vi "Main.vi"(11 "Module Admin":refnum<class "Delacor_lib_QMH_Module Admin.lvclass">) -> ()   [LabVIEW 2019, in "UI.lvlib"]
doc: "This template is based off of the Queued Message Handler design pattern and the Queued Message Handler project template that ships with LabVIEW.\n\nThe main difference is that the queue is private to this module and communication between modules is performed via Broadcast and Request events.\n\nRequest events are wrapped in public API methods and are handled in the Event Handling Loop (EHL) of this VI. Any module can register for Broadcast events sent by this module. The EHL generates messages based on user interface actions.\n\nThe Message Handling Loop (MHL) processes messages generated by the EHL, or by other messages. The messages are string values, so new messages can be added easily to the Message Cases case structure in the MHL. Each message cluster can also provide an optional value for Message Data, which is a variant that can be converted to whatever message-specific data is required.\n_____\nBased on Delacor QMH Project Template 5.0.0.82."
uses:
  UI.lvlib
  <vilib>/Delacor/Delacor QMH/Libraries/Module Admin_class/Delacor_lib_QMH_Module Admin.lvclass
  Module Data--cluster.ctl
  Stop Argument--cluster.ctl
  <vilib>/Delacor/Delacor QMH/Libraries/Message Queue_class/Delacor_lib_QMH_Message Queue.lvclass/Delacor_lib_QMH_Message Queue.ctl
  <vilib>/Delacor/Delacor QMH/Libraries/Module Admin_class/Delacor_lib_QMH_Module Admin.lvclass/Delacor_lib_QMH_Module Admin.ctl
  <vilib>/Delacor/Delacor QMH/Libraries/Message Queue_class/Delacor_lib_QMH_Enqueue Message (Single).vi
  <vilib>/Delacor/Delacor QMH/Libraries/Module Admin_class/Delacor_lib_QMH_Get External Launch.vi
  <vilib>/Utility/error.llb/Error Cluster From Error Code.vi
  <vilib>/ErrorRing/Error Ring.xnode
  <vilib>/Delacor/Delacor QMH/Libraries/Message Queue_class/Delacor_lib_QMH_Message Queue.lvclass
  Mensajes/Messages.lvlib
  Monedas/Monedas.lvlib
  Products/Products.lvlib
  Configuration/Configuration.lvlib
panel:
  out "error out":errorcluster
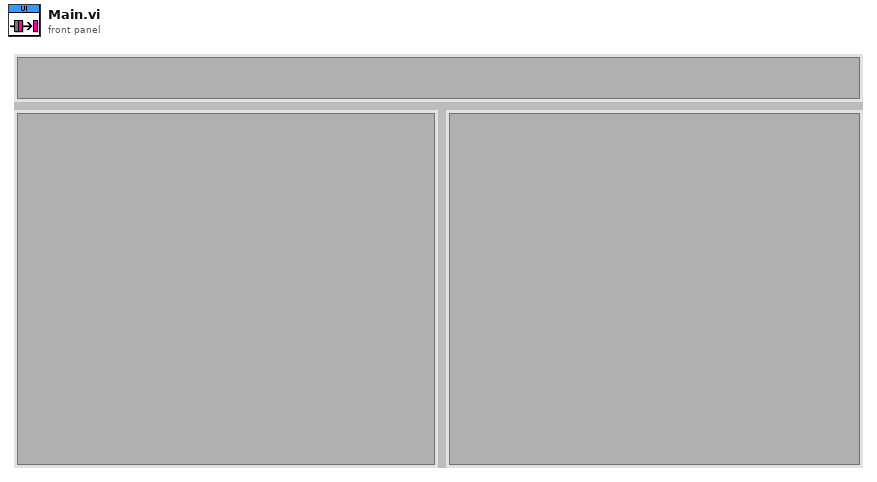
[diagram p1: front panel]
types:
  T1 = typedef "UI.lvlib/Request Events--cluster.ctl" = cluster{"Stop Module":refnum<user-event>, "Show Panel":refnum<user-event>, "Hide Panel":refnum<user-event>, "Get Module Execution Status":refnum<user-event>, "Show Diagram":refnum<user-event>}
  T2 = typedef "Messages.lvlib/Broadcast Events--cluster.ctl" = cluster{"Module Did Init":refnum<user-event>, "Status Updated":refnum<user-event>, "Error Reported":refnum<user-event>, "Module Did Stop":refnum<user-event>, "Update Module Execution Status":refnum<user-event>}
  T3 = typedef "Monedas.lvlib/Broadcast Events--cluster.ctl" = cluster{"Module Did Init":refnum<user-event>, "Status Updated":refnum<user-event>, "Error Reported":refnum<user-event>, "Module Did Stop":refnum<user-event>, "Update Module Execution Status":refnum<user-event>}
  T4 = typedef "Products.lvlib/Broadcast Events--cluster.ctl" = cluster{"Module Did Init":refnum<user-event>, "Status Updated":refnum<user-event>, "Error Reported":refnum<user-event>, "Module Did Stop":refnum<user-event>, "Update Module Execution Status":refnum<user-event>}
  T5 = typedef "Configuration.lvlib/Broadcast Events--cluster.ctl" = cluster{"Module Did Init":refnum<user-event>, "Status Updated":refnum<user-event>, "Error Reported":refnum<user-event>, "Module Did Stop":refnum<user-event>, "Update Module Execution Status":refnum<user-event>}
  T6 = typedef "UI.lvlib/Module Data--cluster.ctl" = cluster{"Status":string}
  T7 = enum32{"invalid lock state", "Not Locked", "Locked (No Password)", "Password-protected"}
  T8 = typedef "UI.lvlib/Stop Argument--cluster.ctl" = cluster{"Origin":string, "Exit via Stop Module Req?":bool, "Wait for Module to stop?":bool}
  T9 = enum32{"Invalid", "Standard", "Closed", "Hidden", "Minimized", "Maximized"}
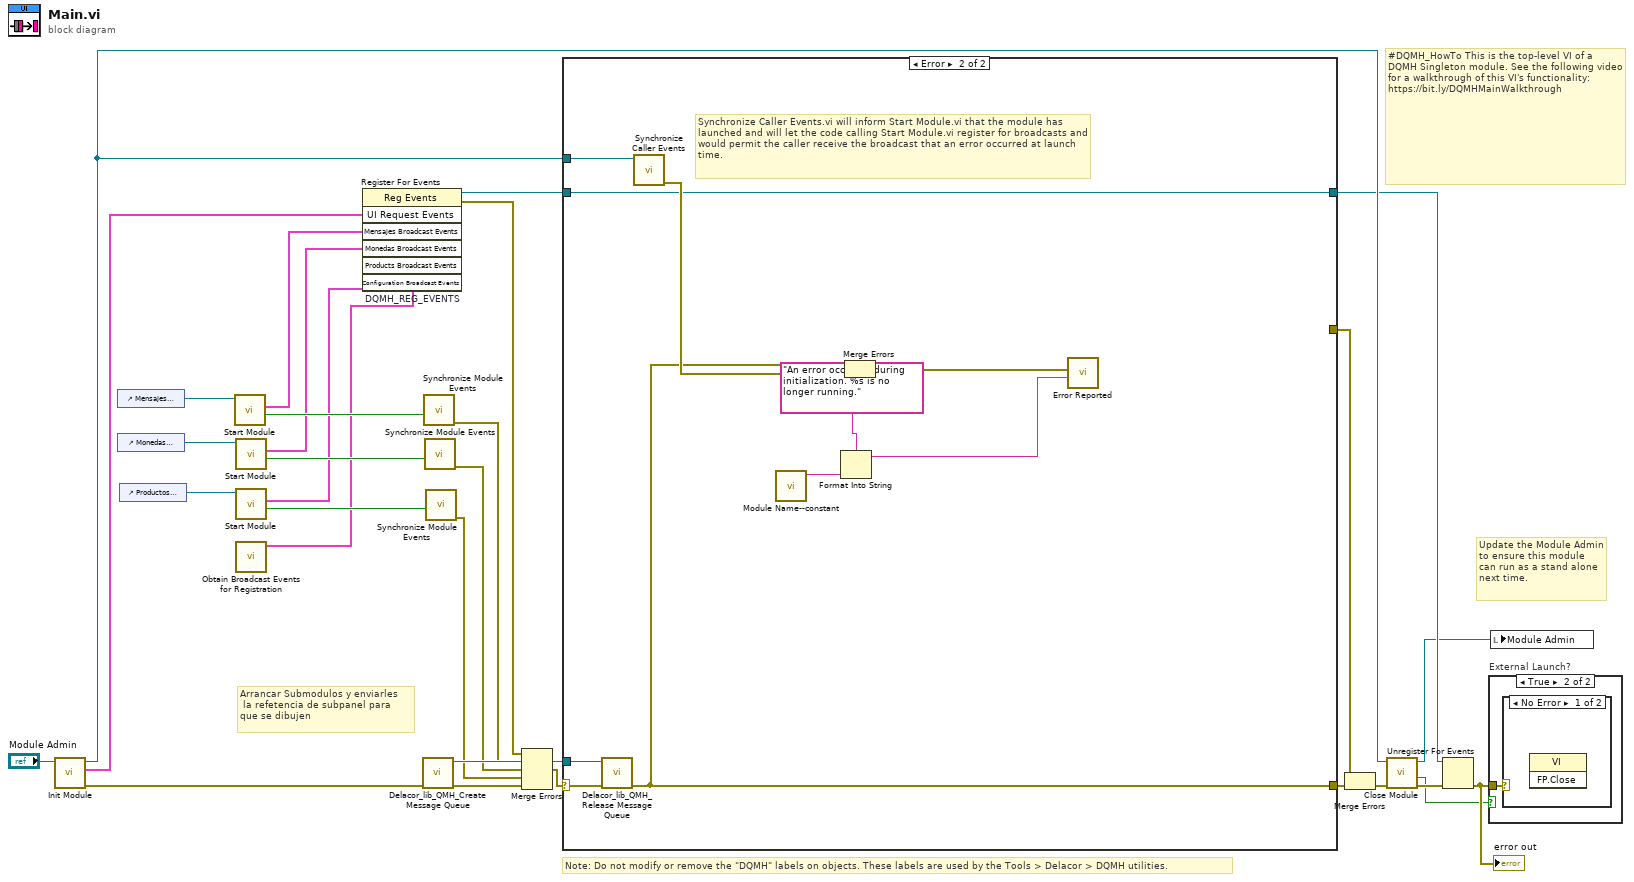
[diagram p0: block diagram]
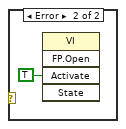
[diagram p3: hidden frame]
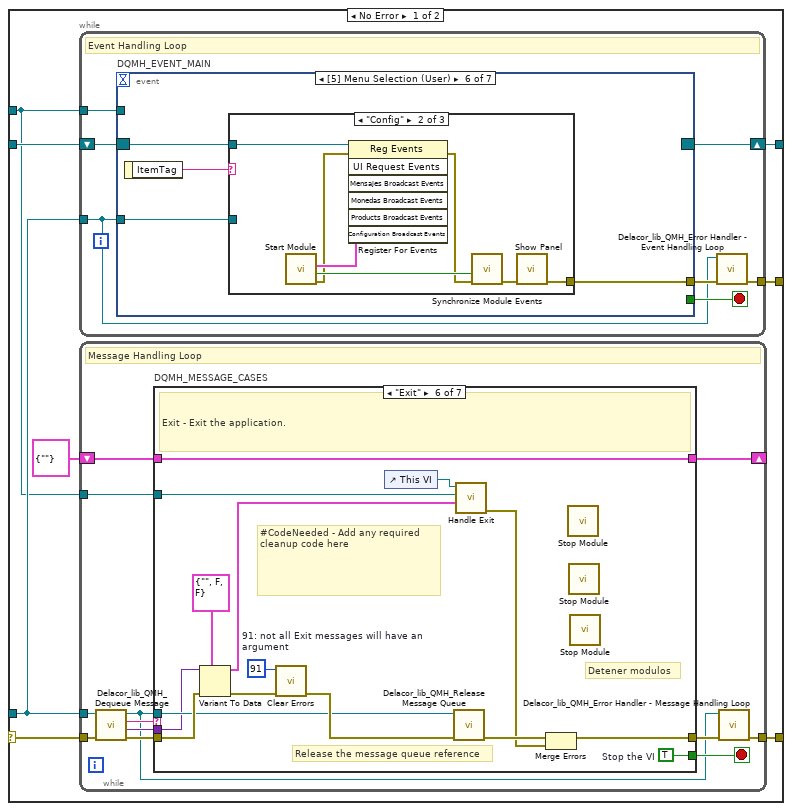
[diagram p4: hidden frame]
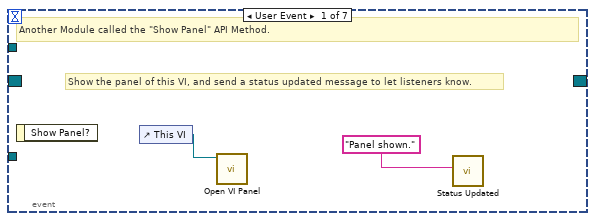
[diagram p5: hidden frame]
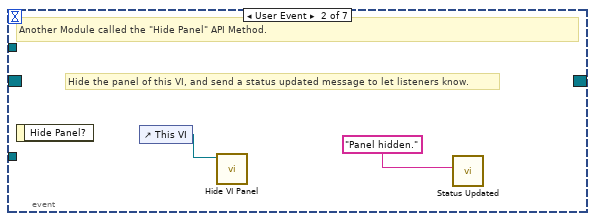
[diagram p6: hidden frame]
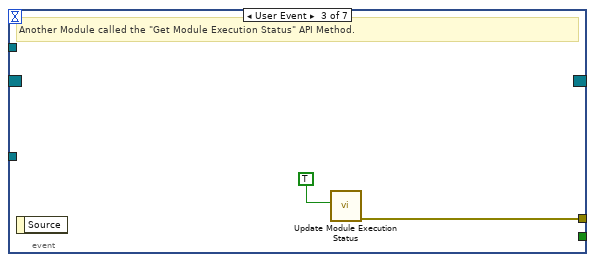
[diagram p7: hidden frame]
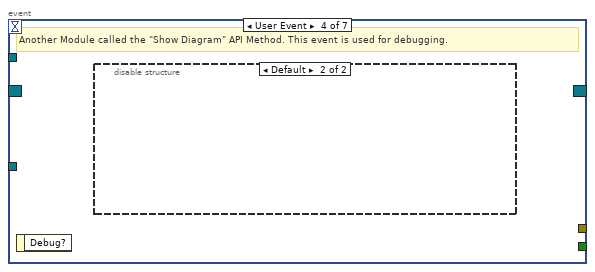
[diagram p8: hidden frame]
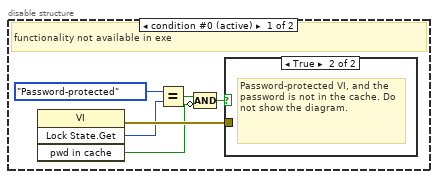
[diagram p9: hidden frame]
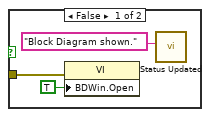
[diagram p10: hidden frame]
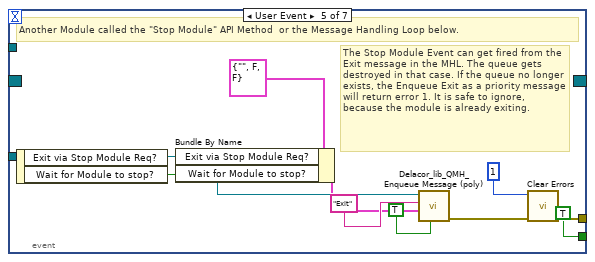
[diagram p11: hidden frame]
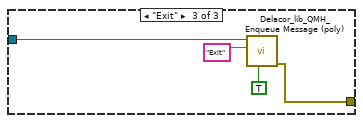
[diagram p13: hidden frame]
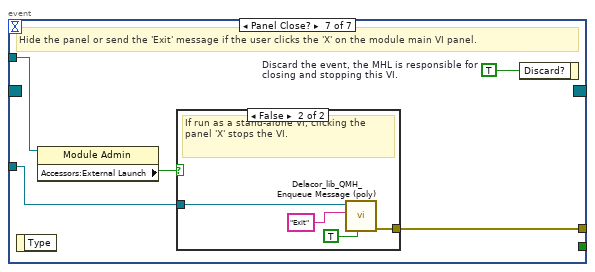
[diagram p14: hidden frame]
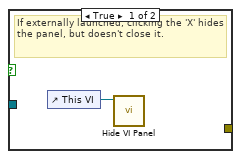
[diagram p15: hidden frame]
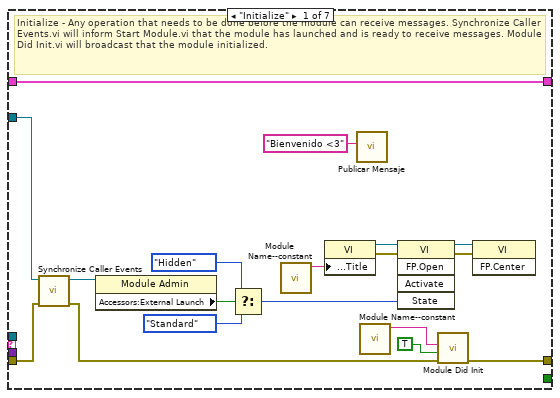
[diagram p16: hidden frame]
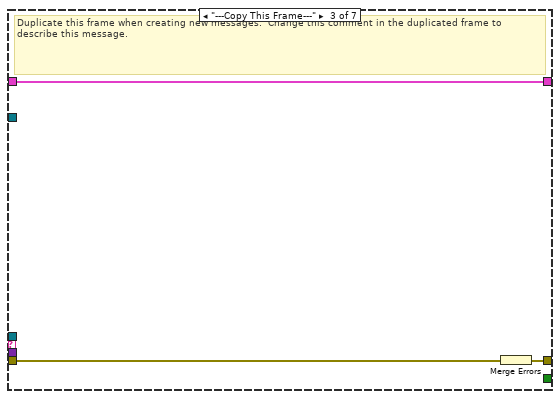
[diagram p18: hidden frame]
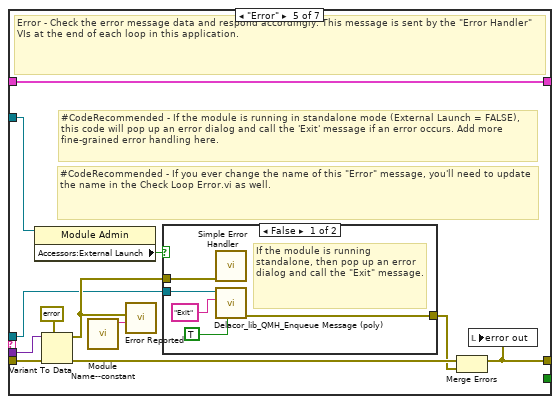
[diagram p20: hidden frame]
diagram:
  # "Arrancar Submodulos y enviarles\n la refetencia de subpanel para \nque se dibujen"
  # "#DQMH_HowTo This is the top-level VI of a DQMH Singleton module. See the following video for a walkthrough of this VI's functionality: https://bit.ly/DQMHMainWalkthrough"
  # "Note: Do not modify or remove the \"DQMH\" labels on objects. These labels are used by the Tools > Delacor > DQMH utilities."
  # "Update the Module Admin to ensure this module can run as a stand alone next time."
  n1 = call "Init Module.vi"("Singleton Module Admin in"="Module Admin") -> ("error out"=w29:errorcluster, "UI Request Events"=w19:T1, "Singleton Module Admin out"=w22:refnum<class "Delacor_lib_QMH_Module Admin.lvclass">)  [unwired: 8 in]
  n2 = control-ref of="Mensajes Subpanel"() -> (w11:refnum<vi>)
  n3 = control-ref of="Monedas Subpanel"() -> (w3:refnum<vi>)
  n4 = control-ref of="Productos Subpanel"() -> (w2:refnum<vi>)
  n5 = call "Start Module.vi"("Mensajes Subpanel"=w11) -> ("Wait for Event Sync?"=w14:bool, "Mensajes Broadcast Events"=w10:T2)  [unwired: 7 in, 2 out]
  n6 = call "Start Module.vi"("Monedas Subpanel"=w3) -> ("Wait for Event Sync?"=w13:bool, "Monedas Broadcast Events"=w9:T3)  [unwired: 7 in, 2 out]
  n7 = call "Start Module.vi"("Productos Subpanel"=w2) -> ("Wait for Event Sync?"=w12:bool, "Products Broadcast Events"=w8:T4)  [unwired: 7 in, 2 out]
  n8 = call "Obtain Broadcast Events for Registration.vi"() -> ("Configuration Broadcast Events"=w1:T5)  [unwired: 9 in, 2 out]
  n9 = register-events "DQMH_REG_EVENTS"(w19, w10, w9, w8, w1) -> (reference out=w20:refnum<event-registration>, error out=w4:errorcluster)  [unwired: 2 in]
  n10 = call <vilib>:"Delacor_lib_QMH_Create Message Queue.vi"("error in (no error)"=w29) -> ("error out"=w24:errorcluster, "Message Queue"=w18:refnum<class "Delacor_lib_QMH_Message Queue.lvclass">)  [unwired: 9 in]
  n11 = call "Synchronize Module Events.vi"("Wait for Event Sync?"=w14) -> ("error out"=w5:errorcluster)  [unwired: 10 in]
  n12 = call "Synchronize Module Events.vi"("Wait for Event Sync?"=w13) -> ("error out"=w6:errorcluster)  [unwired: 10 in]
  n13 = call "Synchronize Module Events.vi"("Wait for Event Sync?"=w12) -> ("error out"=w7:errorcluster)  [unwired: 10 in]
  n14 = Merge Errors(w4, w5, w6, w7, w24) -> (w23:errorcluster)
  n15 = case shown="Error" w23 {
    selector: w23 -> [w36 w182]
    tunnel: [w38 w181] -> w30
    tunnel: [w35 w187] -> w21
    tunnel: w20 -> [w33 w187]
    tunnel: w18 -> [w32 w180]
    tunnel: [w37 _] -> w27
    tunnel: w22 -> [w31 w183]
    frame No Error {
      n16 = while {
        tunnel: w32 -> [w39]
        shift-right: [w42] -> w35
        shift-left: w33 -> [w43]
        tunnel: [w44] -> w37
        tunnel: w31 -> [w40]
        stop <- w41 stop-if-true
        # "Event Handling Loop"
        n17 = event "DQMH_EVENT_MAIN" shown="[5] Menu Selection (User)" {
          selector: w43 -> [_ _ _ _ _ w73 _]
          dyn-events: [_ _ _ _ _ _ _] -> w42
          timeout: _ -> [_ _ _ _ _ _ _]
          tunnel: [_ _ _ _ TRUE ("Discard?") _ _] -> w41
          tunnel: w39 -> [_ _ _ _ w67 w74 w89]
          tunnel: [_ _ w51 _ w70 w72 w91] -> w45
          tunnel: w40 -> [_ _ _ _ _ _ w88]
          event User Event {
            # "Show the panel of this VI, and send a status updated message to let listeners know."
            # "Another Module called the \"Show Panel\" API Method."
            n18 = event-data() -> ()  [unwired: 1 in, 1 out]
            n19 = control-ref of="This VI"() -> (w47:refnum<vi>)
            n20 = call "Open VI Panel.vi"("VI"=w47) -> ()  [unwired: 10 in, 1 out]
            n21 = call "Status Updated.vi"("Status"="Panel shown." ("format string")) -> ()  [unwired: 10 in, 1 out]
          }
          event User Event {
            # "Hide the panel of this VI, and send a status updated message to let listeners know."
            # "Another Module called the \"Hide Panel\" API Method."
            n22 = event-data() -> ()  [unwired: 1 in, 1 out]
            n23 = control-ref of="This VI"() -> (w49:refnum<vi>)
            n24 = call "Hide VI Panel.vi"("VI"=w49) -> ()  [unwired: 10 in, 1 out]
            n25 = call "Status Updated.vi"("Status"="Panel hidden." ("format string")) -> ()  [unwired: 10 in, 1 out]
          }
          event User Event {
            # "Another Module called the \"Get Module Execution Status\" API Method."
            n26 = event-data() -> ()  [unwired: 1 in, 1 out]
            n27 = call "Update Module Execution Status.vi"("Running?"=TRUE) -> ("error out"=w51:errorcluster)  [unwired: 10 in]
          }
          event User Event {
            # "Another Module called the \"Show Diagram\" API Method. This event is used for debugging."
            n28 = event-data() -> ()  [unwired: 1 in, 1 out]
            n29 = disable-structure shown="Default" {
              frame condition #0 (active) {
                # "functionality not available in exe"
                n30 = invoke class="VI" method="Lock State.Get"() -> (error out=w57:errorcluster, "Get Lock State"=w56:T7, "pwd in cache"=w53:bool)  [unwired: 4 in, 1 out]
                n31 = Equal?(x=T7."Password-protected", y=w56) -> (x = y?=w54:bool)
                n32 = Compound Arithmetic op=AND(w54, invert w53) -> (w52:bool)
                n33 = case shown="True" w52 {
                  tunnel: w57 -> [w60 _]
                  frame False {
                    n34 = property class="VI"(error in=w60, "BDWin.Open"=TRUE ("Block Diagram Window:Open")) -> ()  [unwired: 1 in, 2 out]
                    n35 = call "Status Updated.vi"("Status"="Block Diagram shown." ("format string")) -> ()  [unwired: 10 in, 1 out]
                  }
                  frame True {
                    # "Password-protected VI, and the password is not in the cache. Do not show the diagram."
                  }
                }
              }
              frame condition #1 {
              }
            }
          }
          event User Event {
            # "The Stop Module Event can get fired from the Exit message in the MHL. The queue gets destroyed in that case. If the queue no longer exists, the Enqueue Exit as a priority message will return error 1. It is safe to ignore, because the module is already exiting."
            # "Another Module called the \"Stop Module\" API Method  or the Message Handling Loop below."
            n36 = event-data() -> ("Exit via Stop Module Req?"=w63:bool, "Wait for Module to stop?"=w62:bool)  [unwired: 1 in]
            n37 = Bundle By Name(cluster=T8 {"Origin"="", "Exit via Stop Module Req?"=FALSE, "Wait for Module to stop?"=FALSE} ("Stop Argument"), "Exit via Stop Module Req?"=w63, "Wait for Module to stop?"=w62) -> (w61:T8)
            n38 = call-poly <vilib>:"Delacor_lib_QMH_Enqueue Message (poly).vi"("Priority Message? (F)"=TRUE, "Message Data"=w61, "Message"="Exit", "Message Queue in"=w67) -> ("error out"=w71:errorcluster)  [unwired: 6 in, 1 out]
            n39 = call <vilib>:"Clear Errors.vi"("error in (no error)"=w71, "specific error code to clear (0: all)"=1) -> ("error out"=w70:errorcluster)  [unwired: 4 in, 1 out]
          }
          event Menu Selection (User) {
            n40 = event-data() -> ("ItemTag"=w75:string)  [unwired: 1 in]
            n41 = case shown="\"Config\"" w75 {
              tunnel: w74 -> [_ _ w84]
              tunnel: w73 -> [_ w82 _]
              tunnel: [_ w76 w83] -> w72
              frame "False", Default {
              }
              frame "Config" {
                n42 = call "Start Module.vi"() -> ("error out"=w79:errorcluster, "Wait for Event Sync?"=w80:bool, "Configuration Broadcast Events"=w81:T5)  [unwired: 8 in, 1 out]
                n43 = register-events(reference=w82, error in=w79, w81) -> (error out=w78:errorcluster)  [unwired: 4 in, 1 out]
                n44 = call "Synchronize Module Events.vi"("error in (no error)"=w78, "Wait for Event Sync?"=w80) -> ("error out"=w77:errorcluster)  [unwired: 9 in]
                n45 = call "Show Panel.vi"("error in (no error)"=w77) -> ("error out"=w76:errorcluster)  [unwired: 10 in]
              }
              frame "Exit" {
                n46 = call-poly <vilib>:"Delacor_lib_QMH_Enqueue Message (poly).vi"("Priority Message? (F)"=TRUE, "Message"="Exit", "Message Queue in"=w84) -> ("error out"=w83:errorcluster)  [unwired: 7 in, 1 out]
              }
            }
          }
          event Panel Close? {
            w90 = TRUE  # Discard the event, the MHL is responsible for closing and stopping this VI.
            # "Hide the panel or send the 'Exit' message if the user clicks the 'X' on the module main VI panel."
            n47 = event-data() -> ()  [unwired: 1 in, 1 out]
            n48 = property class="Module Admin"(reference=w88) -> ("Accessors:External Launch"=w87:bool)  [unwired: 1 in, 2 out]
            n49 = case shown="False" w87 {
              tunnel: w89 -> [_ w95]
              tunnel: [_ w96] -> w91
              frame True {
                # "If externally launched, clicking the 'X' hides the panel, but doesn't close it."
                n50 = control-ref of="This VI"() -> (w92:refnum<vi>)
                n51 = call "Hide VI Panel.vi"("VI"=w92) -> ()  [unwired: 10 in, 1 out]
              }
              frame False {
                # "If run as a stand-alone VI, clicking the panel 'X' stops the VI."
                n52 = call-poly <vilib>:"Delacor_lib_QMH_Enqueue Message (poly).vi"("Priority Message? (F)"=TRUE, "Message"="Exit", "Message Queue in"=w95) -> ("error out"=w96:errorcluster)  [unwired: 7 in, 1 out]
              }
            }
            n53 = event-data("Discard?"=w90) -> ()  [unwired: 1 in, 1 out]
          }
        }
        n54 = call-dynamic "Delacor_lib_QMH_Error Handler - Event Handling Loop.vi"("error in (no error)"=w45, "Message Queue in"=w39) -> ("dup error in"=w44:errorcluster)  [unwired: 8 in, 1 out]
      }
      n55 = while {
        tunnel: w32 -> [w99]
        shift-right: [w103] -> _
        shift-left: T6 {"Status"=""} ("Data Cluster") -> [w104]
        tunnel: w36 -> [w107]
        tunnel: [w105] -> w38
        tunnel: w31 -> [w97]
        stop <- w102 stop-if-true
        # "Message Handling Loop"
        n56 = call-dynamic "Delacor_lib_QMH_Dequeue Message.vi"("error in (no error)"=w107, "Message Queue in"=w99) -> ("error out"=w106:errorcluster, "Message Data"=w100:variant, "Message"=w101:string, "Message Queue out"=w98:refnum<class "Delacor_lib_QMH_Message Queue.lvclass">)  [unwired: 6 in]
        n57 = case "DQMH_MESSAGE_CASES" shown="\"Exit\"" w101 {
          selector: w101 -> [_ _ _ _ _ _ w167]
          tunnel: w98 -> [_ _ _ _ w137 w159 _]
          tunnel: w106 -> [w124 w128 w131 w133 w144 w165 w169]
          tunnel: [w122 w128 w130 w133 w140 w162 w170] -> w108
          tunnel: w104 -> [w113 w127 w129 w132 w139 w158 w168]
          tunnel: [w113 w127 w129 w132 w139 w158 w168] -> w103
          tunnel: [_ _ _ _ _ w157 _] -> w102
          tunnel: w100 -> [_ _ _ _ w138 w156 _]
          tunnel: w97 -> [w114 _ _ _ w136 w151 _]
          frame "Initialize" {
            # "Initialize - Any operation that needs to be done before the module can receive messages. Synchronize Caller Events.vi will inform Start Module.vi that the module has launched and is ready to receive messages. Module Did Init.vi will broadcast that the module initialized."
            n58 = call "Synchronize Caller Events.vi"("error in (no error)"=w124, "Singleton Module Admin in"=w114) -> ("error out"=w123:errorcluster, "Singleton Module Admin out"=w110:refnum<class "Delacor_lib_QMH_Module Admin.lvclass">)  [unwired: 8 in]
            n59 = property class="Module Admin"(reference=w110) -> ("Accessors:External Launch"=w118:bool)  [unwired: 1 in, 2 out]
            n60 = Select(t=T9."Hidden" ("State"), s=w118, f=T9."Standard" ("State")) -> (s? t:f=w115:T9)
            n61 = call "Module Name--constant.vi"() -> ("Module Name"=w121:string)  [unwired: 11 in]
            n62 = property class="VI"("Front Panel.Title"=w121) -> (reference out=w120:refnum<vi>, error out=w126:errorcluster)  [unwired: 2 in]
            n63 = call "Publicar Mensaje.vi"("Mensaje"="Bienvenido <3") -> ()  [unwired: 10 in, 1 out]
            n64 = call "Module Name--constant.vi"() -> ("Module Name"=w111:string)  [unwired: 11 in]
            n65 = invoke class="VI" method="FP.Open"(reference=w120, error in=w126, "State"=w115) -> (reference out=w119:refnum<vi>, error out=w125:errorcluster)  [unwired: 2 in, 3 out]
            n66 = call "Module Did Init.vi"("error in (no error)"=w123, "Initialized?"=TRUE, "Origin"=w111) -> ("error out"=w122:errorcluster)  [unwired: 8 in]
            n67 = invoke class="VI" method="FP.Center"(reference=w119, error in=w125) -> ()  [unwired: 1 in, 3 out]
          }
          frame "--- Module Specific ---" {
            # "Separator -- The following cases handle messages specific to this Module."
          }
          frame "---Copy This Frame---" {
            # "Duplicate this frame when creating new messages.  Change this comment in the duplicated frame to describe this message."
            n68 = Merge Errors(w131) -> (w130:errorcluster)
          }
          frame "--- Exit and Error Handling---" {
            # "Separator - The following cases handle errors and exit messages."
          }
          frame "Error" {
            # "#CodeRecommended - If you ever change the name of this \"Error\" message, you'll need to update the name in the Check Loop Error.vi as well."
            # "#CodeRecommended - If the module is running in standalone mode (External Launch = FALSE), this code will pop up an error dialog and call the 'Exit' message if an error occurs. Add more fine-grained error handling here."
            # "Error - Check the error message data and respond accordingly. This message is sent by the \"Error Handler\" VIs at the end of each loop in this application."
            n69 = property class="Module Admin"(reference=w136) -> ("Accessors:External Launch"=w135:bool)  [unwired: 1 in, 2 out]
            n70 = Variant To Data(error in=w144, type=errorcluster {"status"=FALSE, "code"=0, "source"=""} ("error constant"), Variant=w138) -> (data=w145:errorcluster, error out=w142:errorcluster)
            n71 = call "Module Name--constant.vi"() -> ("Module Name"=w134:string)  [unwired: 11 in]
            n72 = call "Error Reported.vi"("Additional Information"=w134, "Error"=w145) -> ()  [unwired: 9 in, 1 out]
            n73 = case shown="False" w135 {
              tunnel: [w150 _] -> w141
              tunnel: w137 -> [w148 _]
              tunnel: w145 -> [w149 _]
              frame False {
                # "If the module is running standalone, then pop up an error dialog and call the \"Exit\" message."
                n74 = call <vilib>:"Simple Error Handler.vi"("error in (no error)"=w149) -> ()  [unwired: 4 in, 5 out]
                n75 = call-poly <vilib>:"Delacor_lib_QMH_Enqueue Message (poly).vi"("Priority Message? (F)"=TRUE, "Message"="Exit", "Message Queue in"=w148) -> ("error out"=w150:errorcluster)  [unwired: 7 in, 1 out]
              }
              frame True {
                # "If the module was launched externally, calling the Error Reported broadcast VI is the only action performed by the \"Error\" message. The module's caller can then process the error appropriately."
              }
            }
            n76 = Merge Errors(w142, w141) -> (w140:errorcluster)
            n77 = local write "error out"(w140) -> ()
          }
          frame "Exit" {
            w155 = 91  # 91: not all Exit messages will have an argument
            w157 = TRUE  # Stop the VI
            # "Detener modulos"
            # "Release the message queue reference"
            # "#CodeNeeded - Add any required cleanup code here"
            # "Exit - Exit the application."
            n78 = Variant To Data(error in=w165, type=T8 {"Origin"="", "Exit via Stop Module Req?"=FALSE, "Wait for Module to stop?"=FALSE} ("Stop Argument"), Variant=w156) -> (data=w153:T8, error out=w161:errorcluster)
            n79 = call <vilib>:"Clear Errors.vi"("error in (no error)"=w161, "specific error code to clear (0: all)"=w155) -> ("error out"=w164:errorcluster)  [unwired: 4 in, 1 out]
            n80 = control-ref of="This VI"() -> (w152:refnum<vi>)
            n81 = call-dynamic "Delacor_lib_QMH_Release Message Queue.vi"("error in (no error)"=w164, "Message Queue"=w159) -> ("error out"=w163:errorcluster)  [unwired: 9 in]
            n82 = call "Handle Exit.vi"("Stop Argument"=w153, "Admin in"=w151, "VI reference"=w152) -> ("error out"=w160:errorcluster)  [unwired: 7 in, 1 out]
            n83 = Merge Errors(w163, w160) -> (w162:errorcluster)
            n84 = call "Stop Module.vi"() -> ()  [unwired: 11 in, 1 out]
            n85 = call "Stop Module.vi"() -> ()  [unwired: 11 in, 1 out]
            n86 = call "Stop Module.vi"() -> ()  [unwired: 11 in, 1 out]
          }
          frame Default {
            # "'Default' case only runs if there is a message that isn't defined in any of the other cases.  Output a programming error."
            n87 = call "Module Name--constant.vi"() -> ("Module Name"=w166:string)  [unwired: 11 in]
            n88 = xnode "Error Ring"("parameter 0"=w167, "parameter 1"=w166) -> ("error out"=w171:errorcluster)
            n89 = Merge Errors(w169, w171) -> (w170:errorcluster)
          }
        }
        n90 = call-dynamic "Delacor_lib_QMH_Error Handler - Message Handling Loop.vi"("error in (no error)"=w108, "Message Queue in"=w98) -> ("dup error in"=w105:errorcluster)  [unwired: 8 in, 1 out]
      }
    }
    frame Error {
      # "Synchronize Caller Events.vi will inform Start Module.vi that the module has launched and will let the code calling Start Module.vi register for broadcasts and would permit the caller receive the broadcast that an error occurred at launch time."
      n91 = call-dynamic "Delacor_lib_QMH_Release Message Queue.vi"("error in (no error)"=w182, "Message Queue"=w180) -> ("error out"=w181:errorcluster)  [unwired: 9 in]
      n92 = call "Synchronize Caller Events.vi"("Singleton Module Admin in"=w183) -> ("error out"=w188:errorcluster)  [unwired: 9 in, 1 out]
      n93 = call "Module Name--constant.vi"() -> ("Module Name"=w186:string)  [unwired: 11 in]
      n94 = Format Into String(format string="An error occurred during initialization. %s is no longer running.", w186) -> (resulting string=w184:string)  [unwired: 2 in, 1 out]
      n95 = Merge Errors(w181, w188) -> (w189:errorcluster)
      n96 = call "Error Reported.vi"("Additional Information"=w184, "Error"=w189) -> ()  [unwired: 9 in, 1 out]
    }
  }
  n97 = Merge Errors(w27, w30) -> (w26:errorcluster)
  n98 = call "Close Module.vi"("error in (no error)"=w26, "Module Admin in"=w22) -> ("error out"=w28:errorcluster, "External Launch"=w15:bool, "Module Admin out"=w16:refnum<class "Delacor_lib_QMH_Module Admin.lvclass">)  [unwired: 7 in]
  n99 = Unregister For Events(event registration refnum=w21, error in=w28) -> (error out=w25:errorcluster)
  "error out" <- w25
  n100 = case "External Launch?" shown="True" w15 {
    tunnel: w25 -> [_ w190]
    frame False {
    }
    frame True {
      n101 = case shown="No Error" w190 {
        frame No Error {
          n102 = invoke class="VI" method="FP.Close"() -> ()  [unwired: 3 in, 3 out]
        }
        frame Error {
          n103 = invoke class="VI" method="FP.Open"("Activate"=TRUE ("Activate?")) -> ()  [unwired: 4 in, 5 out]
        }
      }
    }
  }
  n104 = local write "Module Admin"(w16) -> ()
